vi "AutomatedStart_Flo.vi"() -> ()   [LabVIEW 2014]
uses:
  <vilib>/userdefined/High Color/nirio_resource_hc.ctl
  TriggerChannel.ctl
  <vilib>/FPGAPlugInAG/PCI-7813R/niLvFpga_Open_PCI-7813R.vi
  <vilib>/rvi/interface/nirviOpenFPGA/nirviOpenFPGA.xnode
  FPGA Bitfiles/W7XBolo2017_FPGATarget_fmain2014_9xlV3GyHFfo.lvbitx
  f_main_2014.vi
panel:
  out "Operation Watchdog":bool
  out "No. of Software Triggers \ndetected":dbl
  out "No. of Hardware Triggers \ndetected":dbl
  out "Autmated Start Loop Counter \n(Increasing every 1s)":i32
  out "Timeout ? \n(1s-10s?)":bool
  out "Hardware Trigger \ndetected":bool
  in  "Software Trigger\n(Switch until released)":bool
  in  "Stopp Button":bool
  # "Automated Start W7-X Bolometer DAQ"
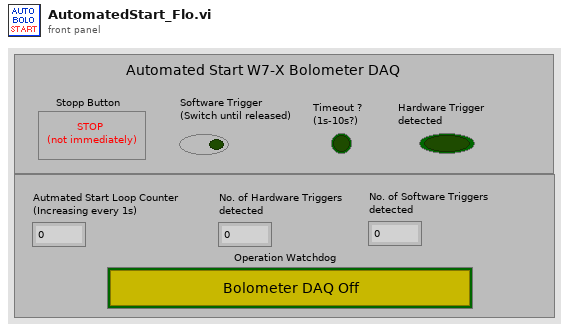
[diagram p1: front panel]
types:
  T1 = typedef "TriggerChannel.ctl" = enum16{"board0 (broken)", "board1 (t = -60sec)", "board2 (t = 0sec)"}
  T2 = enum32{"Invalid", "Standard", "Closed", "Hidden", "Minimized", "Maximized"}
  T3 = typedef "nirio_resource_hc.ctl" = tag
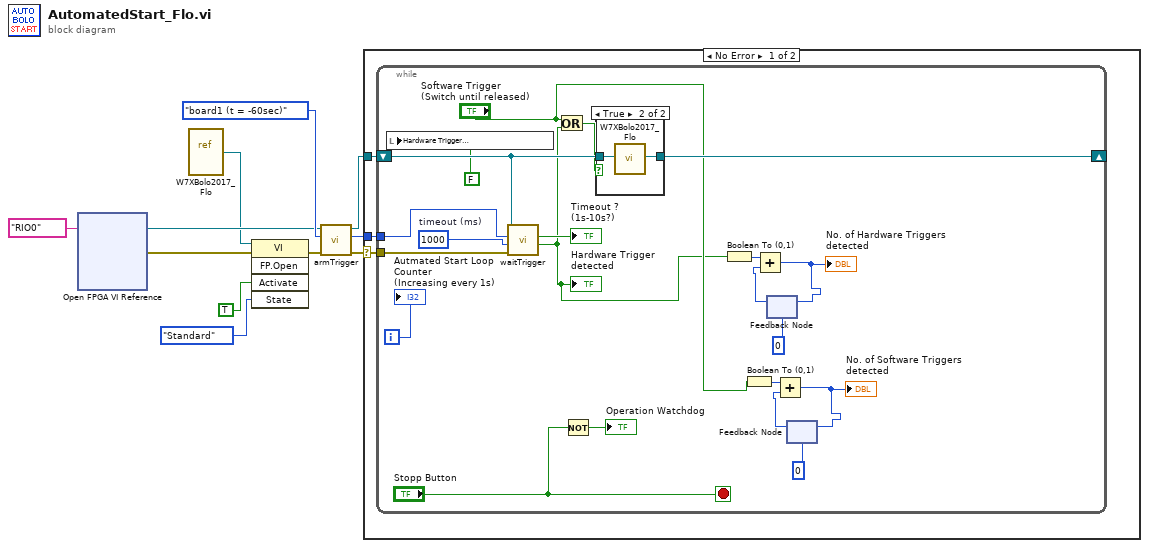
[diagram p0: block diagram]
diagram:
  n1 = xnode "Open FPGA VI Reference"("resource name"=T3 "RIO0") -> ("FPGA VI Reference Out"=w4:refnum<k20>, "error out"=w8:errorcluster)  [unwired: 1 in]
  n2 = vi-ref "W7XBolo2017_Flo.vi"() -> (w1:refnum<vi>)
  n3 = invoke class="VI" method="FP.Open"(reference=w1, error in=w8, "Activate"=TRUE ("Activate?"), "State"=T2."Standard") -> (error out=w7:errorcluster)  [unwired: 1 in, 4 out]
  n4 = call "armTrigger.vi"("error in (no error)"=w7, "Trigger default: board0 (t = 0)"=TriggerChannel."board1 (t = -60sec)", "Refnum in"=w4) -> ("error out"=w6:errorcluster, "IRQ"=w2:i32, "Refnum out"=w3:refnum<k20>)  [unwired: 6 in]
  n5 = case shown="No Error" w6 {
    selector: w6 -> [w12 _]
    tunnel: w3 -> [w14 _]
    tunnel: w2 -> [w13 _]
    frame No Error {
      n6 = while {
        shift-right: [w34] -> _
        shift-left: w14 -> [w35]
        tunnel: w13 -> [w32]
        tunnel: w12 -> [w31]
        i -> [w28]
        stop <- "Stopp Button" stop-if-true
        w33 = 1000  # timeout (ms)
        n7 = local write "Hardware Trigger \ndetected"(FALSE) -> ()
        n8 = call "waitTrigger.vi"("error in (no error)"=w31, "timeout (ms) default: 10s"=w33, "IRQ"=w32, "Refnum in"=w35) -> ("Boolean"=w17:bool, "Timed Out"=→"Timeout ? \n(1s-10s?)":bool)  [unwired: 4 in, 2 out]
        "Hardware Trigger \ndetected" <- w17
        n9 = Or(x="Software Trigger\n(Switch until released)", y=w17) -> (x .or. y?=w23:bool)
        n10 = Not(x="Stopp Button") -> (.not. x?=→"Operation Watchdog":bool)
        n11 = case shown="True" w23 {
          tunnel: w35 -> [w36 w38]
          tunnel: [w36 w37] -> w34
          frame False {
          }
          frame True {
            n12 = call "W7XBolo2017_Flo.vi"("FPGA VI Reference In"=w38) -> ("FPGA VI Reference Out"=w37:refnum<k20>)
          }
        }
        n13 = Boolean To (0,1)(Boolean=w17) -> (0, 1=w26:i16)
        n14 = Boolean To (0,1)(Boolean="Software Trigger\n(Switch until released)") -> (0, 1=w21:i16)
        n15 = feedback #1(i16 0) -> (w27:i16)
        n16 = Add(x=w26, y=w27) -> (x+y=w24:i16)
        "No. of Hardware Triggers \ndetected" <- w24
        n17 = feedback-in #1(w24) -> ()
        n18 = feedback #2(i16 0) -> (w22:i16)
        n19 = Add(x=w21, y=w22) -> (x+y=w19:i16)
        "No. of Software Triggers \ndetected" <- w19
        n20 = feedback-in #2(w19) -> ()
        "Autmated Start Loop Counter \n(Increasing every 1s)" <- w28
      }
    }
    frame Error {
    }
  }
